vi "avaliaPertoDaParede.vi"(8 "Distância":dbl format="%#_13g", 9 "Y":dbl format="%#_13g", 10 "X":dbl format="%#_13g", 11 "IA State":T2={"our_robots"=[], "enemy_robots"=[], "balls"=[], "geometry"={"field_length"=0, "field_width"=0, "goal_width"=0, "goal_depth"=0, "center_circle_radius"=0, "defense_width"=0, "defense_depth"=0, "free_kick_from_defense_dist"=0, "penalty_spot_from_field_line_dist"=0, "penalty_line_from_spot_dist"=0, "half_moon_depth"=0, "half_moon_width"=0}, "IA Judge"={"stage"="", "command"="", "our_goalie_id"=0.0, "enemy_goalie_id"=0.0, "command enum"=enum."Halt", "Time"=enum."Azul"}, "Received Timestamp"=timestamp(0 s since 1904-01-01), "Events"={"Touch"=FALSE, "id touch"=0.0, "Ball out of \nVision"=FALSE, "Ball inside \nGoalie area"=FALSE, "Robot not responding"=FALSE, "Robots responding status"=[1.0, 1.0, 1.0, 1.0, 1.0, 1.0], "Enemy Ball \nPossession"=FALSE, "Id ini Possession"=0.0, "Ball Possesion"=FALSE, "Id Possesion"=0.0, "Ball at\nour goal side"=FALSE, "Ball at\ntouchline"=FALSE, "Ball at\nenemy goal side"=FALSE}}) -> (2 "Enum":T1(ring), 3 "Perto de parede?":bool=TRUE)   [LabVIEW 2018]
doc: "Função que avalia se um objeto está perto das paredes ou não, e retorna qual parede."
uses:
  Core/AI Input.ctl
  Core/AI Robot.ctl
  Intel/Functions Enum.ctl
  Intel/AttackerStates.ctl
  Path Planning/RRT/PathDests.ctl
  Path Planning/RRT/PathDest.ctl
  Core/AI Ball.ctl
  Core/Field Size.ctl
  Core/AI Judge.ctl
  Intel/Command Enum.ctl
  Util/Events/Events.ctl
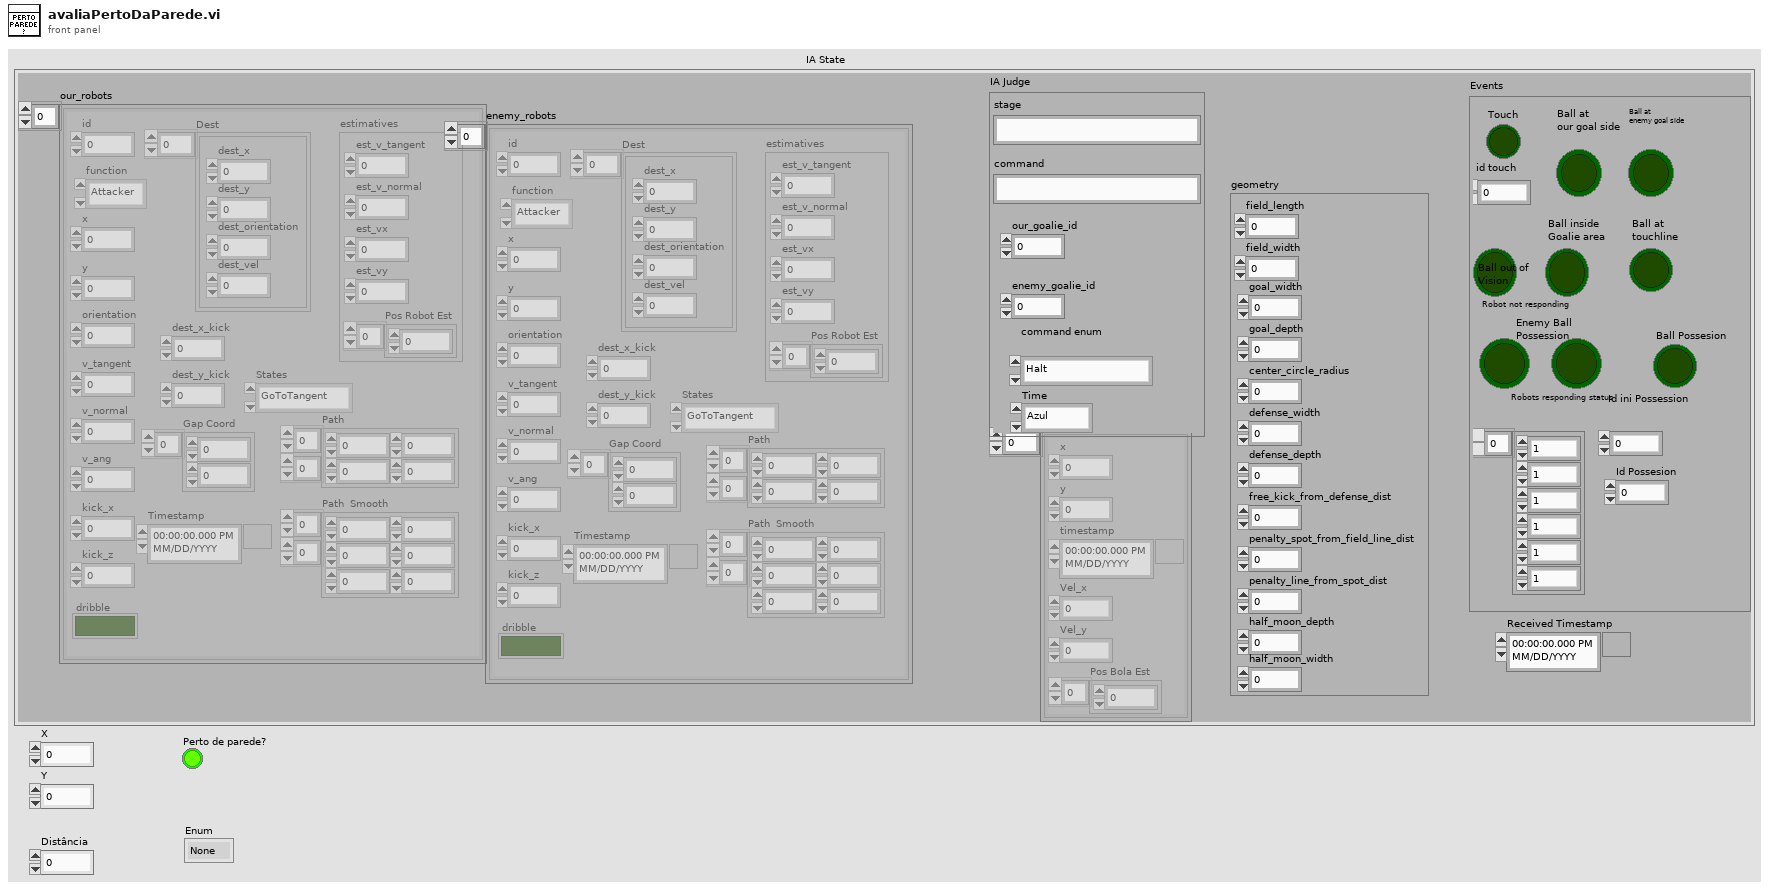
[diagram p1: front panel]
types:
  T1 = enum16{"None", "Frente", "Trás", "Cima", "Baixo"}
  T2 = typedef "AI Input.ctl" = cluster{"our_robots":T3[], "enemy_robots":T3[], "balls":T8[], "geometry":T9, "IA Judge":T10, "Received Timestamp":timestamp, "Events":T12}
  T3 = typedef "AI Robot.ctl" = cluster{"id":u32, "function":T4, "x":dbl, "y":dbl, "orientation":dbl, "v_tangent":dbl, "v_normal":dbl, "v_ang":dbl, "kick_x":dbl, "kick_z":dbl, "dribble":bool, "Timestamp":timestamp, "estimatives":cluster{"est_v_tangent":dbl, "est_v_normal":dbl, "est_vx":dbl, "est_vy":dbl, "Pos Robot Est":dbl[]}, "dest_x_kick":dbl, "dest_y_kick":dbl, "Gap Coord":dbl[], "States":T5, "Path ":dbl[][], "Path  Smooth":dbl[][], "Dest":T6}
  T4 = typedef "Functions Enum.ctl" = enum16{"Attacker", "Goalie", "Defender", "Striker", "Goto 0", "Dummy", "Kicker", "ZigZag"}
  T5 = typedef "AttackerStates.ctl" = enum16{"Pass", "GoToTangent", "BallGetting", "GoToKick", "Rotate anti-clockwise", "Rotate Clockwise", ""}
  T6 = typedef "PathDests.ctl" = T7[]
  T7 = typedef "PathDest.ctl" = cluster{"dest_x":dbl, "dest_y":dbl, "dest_orientation":dbl, "dest_vel":dbl}
  T8 = typedef "AI Ball.ctl" = cluster{"x":dbl, "y":dbl, "timestamp":timestamp, "Vel_x":dbl, "Vel_y":dbl, "Pos Bola Est":dbl[]}
  T9 = typedef "Field Size.ctl" = cluster{"field_length":u32, "field_width":u32, "goal_width":u32, "goal_depth":u32, "center_circle_radius":u32, "defense_width":u32, "defense_depth":u32, "free_kick_from_defense_dist":u32, "penalty_spot_from_field_line_dist":u32, "penalty_line_from_spot_dist":u32, "half_moon_depth":u32, "half_moon_width":u32}
  T10 = typedef "AI Judge.ctl" = cluster{"stage":string, "command":string, "our_goalie_id":dbl, "enemy_goalie_id":dbl, "command enum":T11, "Time":enum16{"Azul", "Amarelo"}}
  T11 = typedef "Command Enum.ctl" = enum16{"Halt", "Stop", "Force Start", "PKA Normal Start", "Prepare Kickoff Ally", "PKE Normal Start", "Prepare Kickoff Enemy", "Prepare Penalty Ally", "PPA Normal Start", "Prepare Penalty Enemy", "PPE Normal Start", "Ball Placement Enemy Up", "Ball Placement Enemy Down", "Ball Placement Ally Up", "Ball Placement Ally Mid", "Ball Placement Ally Down", "Indirect Free Enemy", "Indirect Free Ally", "Timeout Enemy", "Timeout Ally", "Goal Enemy", "Goal Ally", "Normal Half Time", "Extra Time Break", "Extra Half Time", "None", "Post Game"}
  T12 = typedef "Events.ctl" = cluster{"Touch":bool, "id touch":dbl, "Ball out of \nVision":bool, "Ball inside \nGoalie area":bool, "Robot not responding":bool, "Robots responding status":dbl[], "Enemy Ball \nPossession":bool, "Id ini Possession":dbl, "Ball Possesion":bool, "Id Possesion":dbl, "Ball at\nour goal side":bool, "Ball at\ntouchline":bool, "Ball at\nenemy goal side":bool}
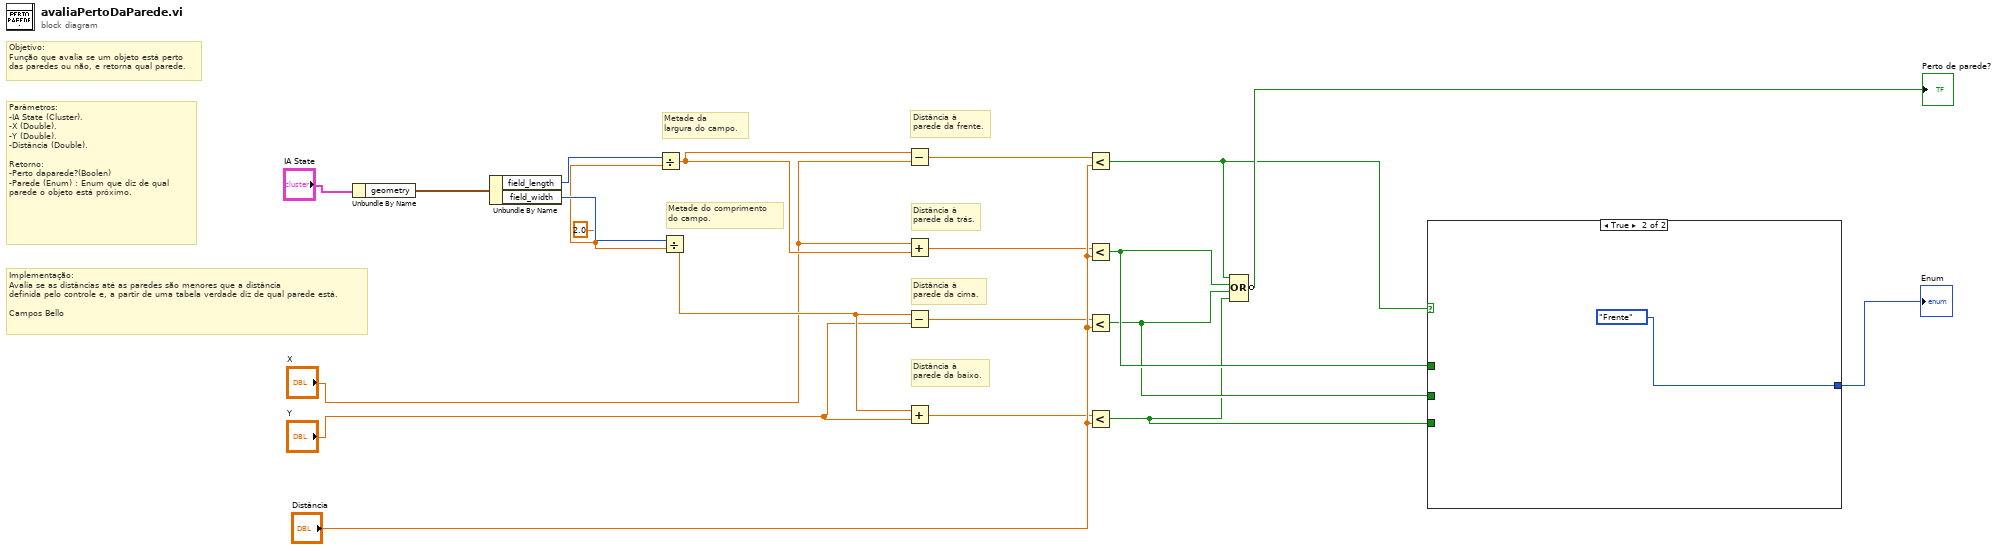
[diagram p0: block diagram]
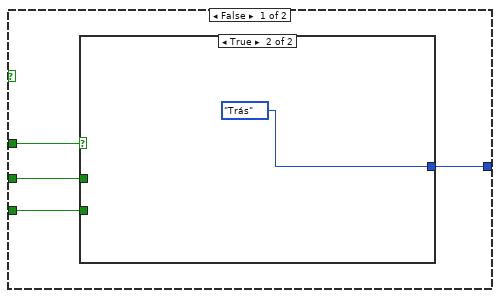
[diagram p2: hidden frame]
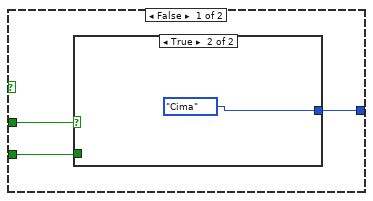
[diagram p3: hidden frame]
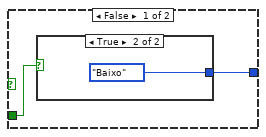
[diagram p4: hidden frame]
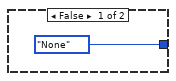
[diagram p5: hidden frame]
diagram:
  w16 = 2.0 ("y")
  # "Parâmetros:\n-IA State (Cluster).\n-X (Double).\n-Y (Double).\n-Distância (Double).\n\nRetorno:\n-Perto daparede?(Boolen)\n-Parede (Enum) : Enum que diz de qual parede o objeto está próximo."
  # "Implementação:\nAvalia se as distâncias até as paredes são menores que a distância\ndefinida pelo controle e, a partir de uma tabela verdade diz de qual parede está.\n\nCampos Bello"
  # "Objetivo:\nFunção que avalia se um objeto está perto\ndas paredes ou não, e retorna qual parede."
  # "Distância à\nparede da baixo."
  # "Distância à\nparede da cima."
  # "Distância à\nparede da trás."
  # "Distância à\nparede da frente."
  # "Metade do comprimento\ndo campo."
  # "Metade da\nlargura do campo."
  n1 = Unbundle By Name("IA State") -> ("geometry"=w19:T9)
  n2 = Unbundle By Name(w19) -> ("field_length"=w18:u32, "field_width"=w17:u32)
  n3 = Divide(x=w18, y=w16) -> (x/y=w15:dbl)
  n4 = Divide(x=w17, y=w16) -> (x/y=w14:dbl)
  n5 = Subtract(x=w15, y="X") -> (x-y=w12:dbl)
  n6 = Add(x="X", y=w15) -> (x+y=w11:dbl)
  n7 = Subtract(x=w14, y="Y") -> (x-y=w10:dbl)
  n8 = Add(x=w14, y="Y") -> (x+y=w9:dbl)
  n9 = Less?(x=w12, y="Distância") -> (x < y?=w7:bool)
  n10 = Less?(x=w11, y="Distância") -> (x < y?=w6:bool)
  n11 = Less?(x=w10, y="Distância") -> (x < y?=w5:bool)
  n12 = Less?(x=w9, y="Distância") -> (x < y?=w4:bool)
  n13 = Compound Arithmetic op=OR(w7, w6, w5, w4) -> (invert →"Perto de parede?":bool)
  n14 = case shown="True" w7 {
    tunnel: w6 -> [w24 _]
    tunnel: w5 -> [w23 _]
    tunnel: w4 -> [w22 _]
    tunnel: [w21 T1."Frente" ("Enum")] -> w3
    frame False {
      n15 = case shown="True" w24 {
        tunnel: w23 -> [w27 _]
        tunnel: w22 -> [w26 _]
        tunnel: [w25 T1."Trás" ("Enum")] -> w21
        frame False {
          n16 = case shown="True" w27 {
            tunnel: w26 -> [w29 _]
            tunnel: [w28 T1."Cima" ("Enum")] -> w25
            frame False {
              n17 = case shown="True" w29 {
                tunnel: [T1."None" ("Enum") T1."Baixo" ("Enum")] -> w28
                frame False {
                }
                frame True {
                }
              }
            }
            frame True {
            }
          }
        }
        frame True {
        }
      }
    }
    frame True {
    }
  }
  "Enum" <- w3
